vi "Moving Avg.vi"(2 "new measurement":dbl) -> (0 "mean":dbl format="%0.2f")   [LabVIEW 2011]
uses:
  <vilib>/Analysis/NI_AALBase.lvlib
panel:
  out "output array":dbl[](array[numeric])
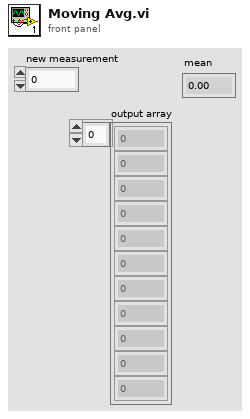
[diagram p1: front panel]
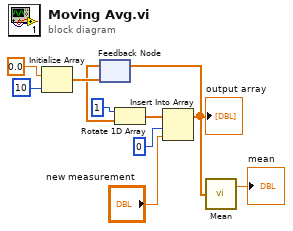
[diagram p0: block diagram]
diagram:
  n1 = Initialize Array(0.0 ("element"), 10 ("dimension size")) -> (w8:dbl[])
  n2 = feedback #1(w8) -> (w7:dbl[])
  n3 = Rotate 1D Array(1:w7, 2:1 ("n")) -> (0:w5:dbl[])
  n4 = Insert Into Array(array=w5, index=0, new element="new measurement") -> (w3:dbl[])
  "output array" <- w3
  n5 = feedback-in #1(w3) -> ()
  n6 = call <vilib>:"Mean.vi"("X"=w3) -> ("mean"=→"mean":dbl)  [unwired: 1 out]
